vi "測試環境.vi"() -> ()   [LabVIEW 2021]
panel:
  in  "電源":bool
  in  "停止":bool
  out "管路電子閥":bool(xcontrol)
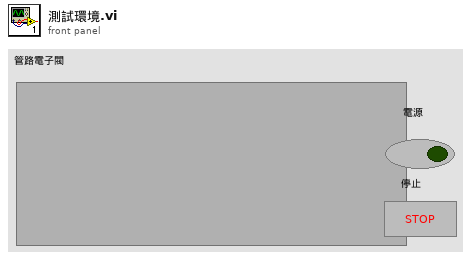
[diagram p1: front panel]
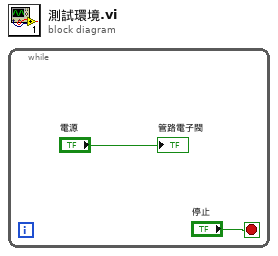
[diagram p0: block diagram]
diagram:
  n1 = while {
    stop <- "停止" stop-if-true
    "管路電子閥" <- "電源"
  }
